vi "SOC detect.vi"(10 "Vmeasure":dbl format="%#_13g") -> (2 "testresult":bool, 3 "SOC":string)   [LabVIEW 2020]
uses:
  Param_Sys.vi
panel:
  in  "30%":bool=TRUE
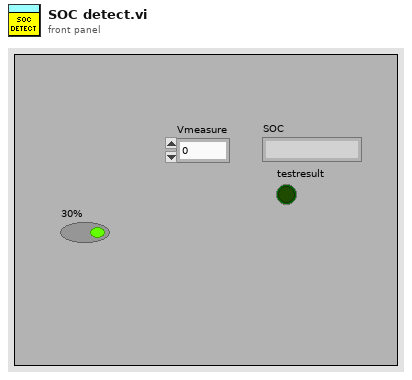
[diagram p1: front panel]
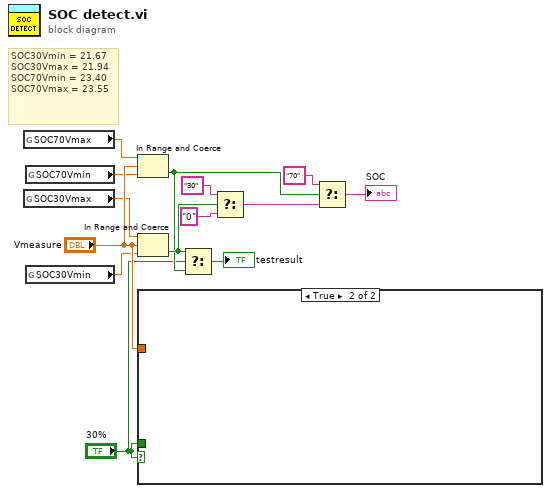
[diagram p0: block diagram]
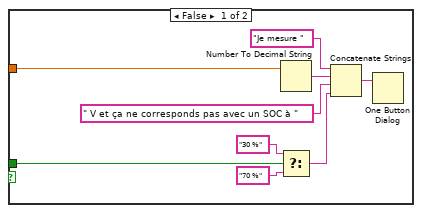
[diagram p2: hidden frame]
diagram:
  # "SOC30Vmin = 21.67\nSOC30Vmax = 21.94\nSOC70Vmin = 23.40\nSOC70Vmax = 23.55"
  n1 = global read "Param_Sys.vi" "SOC70Vmax"() -> (w9:dbl)
  n2 = global read "Param_Sys.vi" "SOC30Vmax"() -> (w3:dbl)
  n3 = global read "Param_Sys.vi" "SOC70Vmin"() -> (w4:dbl)
  n4 = global read "Param_Sys.vi" "SOC30Vmin"() -> (w2:dbl)
  n5 = In Range and Coerce(upper limit=w9, x="Vmeasure", lower limit=w4) -> (In Range?=w7:bool)  [unwired: 1 out]
  n6 = In Range and Coerce(upper limit=w3, x="Vmeasure", lower limit=w2) -> (In Range?=w8:bool)  [unwired: 1 out]
  n7 = case shown="True" "30%" {
    tunnel: "Vmeasure" -> [w22 _]
    tunnel: "30%" -> [w19 _]
    frame False {
      n8 = Number To Decimal String(number=w22) -> (decimal integer string=w21:string)  [unwired: 1 in]
      n9 = Select(t="30 %" ("message"), s=w19, f="70 %" ("message")) -> (s? t:f=w16:string)
      n10 = Concatenate Strings("Je mesure " ("message"), w21, " V et ça ne corresponds pas avec un SOC à " ("string"), w16) -> (w15:string)
      n11 = One Button Dialog(message=w15) -> ()  [unwired: 1 in, 1 out]
    }
    frame True {
    }
  }
  n12 = Select(t=w8, s="30%", f=w7) -> (s? t:f=→"testresult":bool)
  n13 = Select(t="30", s=w8, f="0") -> (s? t:f=w12:string)
  n14 = Select(t="70", s=w7, f=w12) -> (s? t:f=→"SOC":string)
